vi "GrabToTrackerAndQueue(LostFramesSupport).vi"(0 "IMAQ Refnum in":refnum<k11>, 1 "Tracking enabled?":bool, 2 "Framerate":i32, 3 "QTrk Instance":T6, 4 "ROIs":cluster{"X":i32, "Y":i32}[](array[cluster]), 6 "stop":refnum<vi>, 7 "Type":T5, 8 "Send to queue?":bool, 9 "#ROI":i32, 10 "Output Queue":refnum<queue>, 12 "ResultManager":T4, 13 "ROI Size":cluster{"X":i32, "Y":i32}) -> ()   [LabVIEW 2011]
uses:
  qtrk/QTrkLVBinding/QTrkInstance.ctl
  Main/Typedefs/CmdEnum_CameraFrameType.ctl
  qtrk/QTrkLVBinding/ResultManagerInstance.ctl
  Main/Typedefs/CmdData_NewFrame.ctl
  <vilib>/vision/Image Controls.llb/IMAQ Image.ctl
  Main/Motors/MotorPosType.ctl
  Main/Typedefs/XYf.ctl
  qtrk/QTrkLVBinding/QTrkDLL.vi
  Main/GlobalVariables.vi
panel:
  out "Current Position":T1
  out "widths":u32[](array[numeric])
  out "Preloaded timestamps":u32[](array[numeric])
  in  "Stop2":bool
  in  "Show image?":bool
  out "Image":T3(plugin-control)
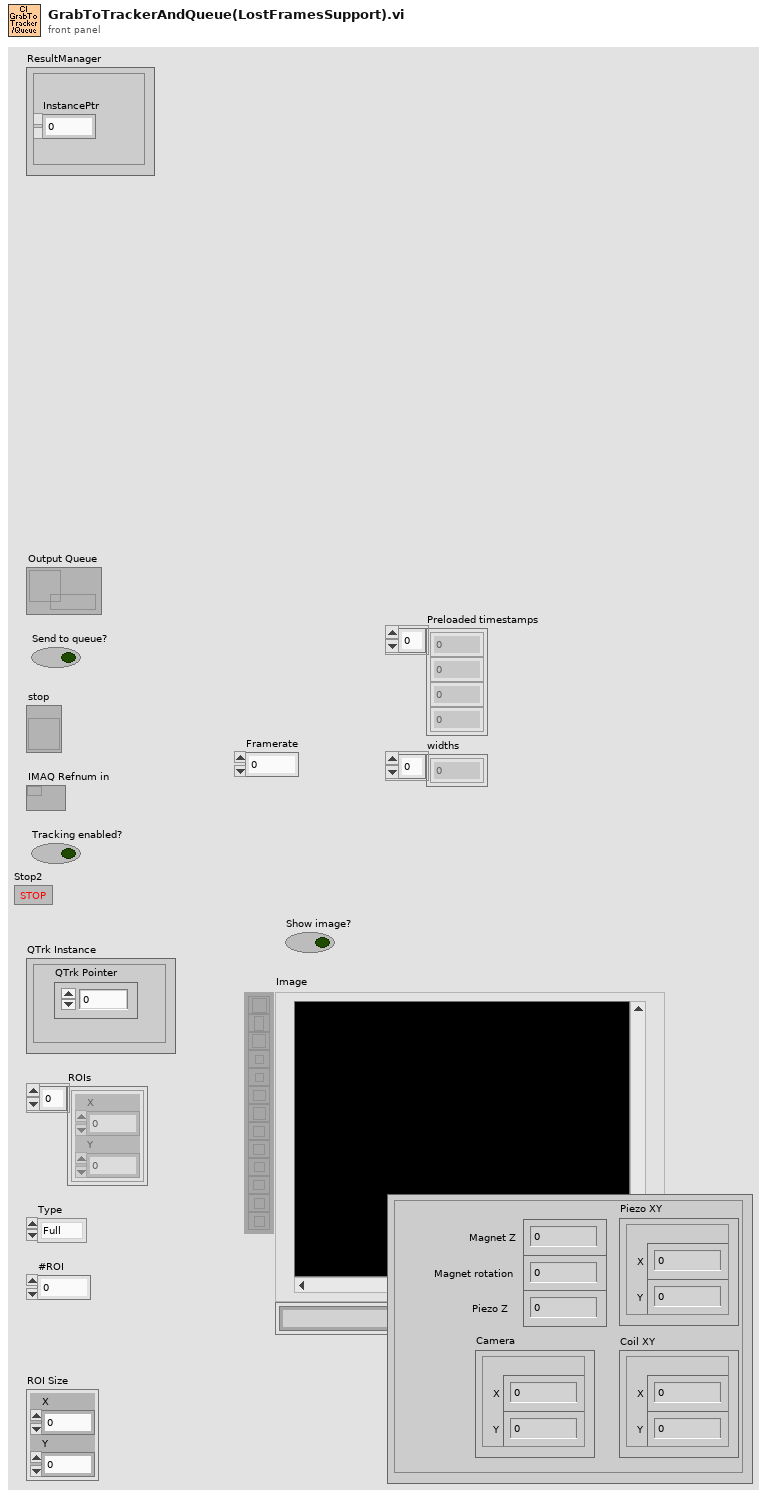
[diagram p1: front panel]
types:
  T1 = typedef "MotorPosType.ctl" = cluster{"Magnet Z":dbl, "Magnet rotation":dbl, "Camera":T2, "Piezo XY":T2, "Piezo Z":dbl, "Coil XY":T2}
  T2 = typedef "XYf.ctl" = cluster{"X":sgl, "Y":sgl}
  T3 = typedef "IMAQ Image.ctl" = refnum<image>
  T4 = typedef "ResultManagerInstance.ctl" = cluster{"InstancePtr":u64}
  T5 = typedef "CmdEnum_CameraFrameType.ctl" = enum16{"Full", "HardwareROI", "EndGrabMarker"}
  T6 = typedef "QTrkInstance.ctl" = cluster{"QTrk Pointer":u64}
  T7 = typedef "MotorStateType.ctl" = cluster{"Enabled?":bool, "Current Position":T1, "Update counter":i32}
  T8 = typedef "CmdData_NewFrame.ctl" = cluster{"Buffer Image":T3, "Frame #":i32, "Hardware ROI Index":i32, "Timestamp":dbl, "Type":T5}
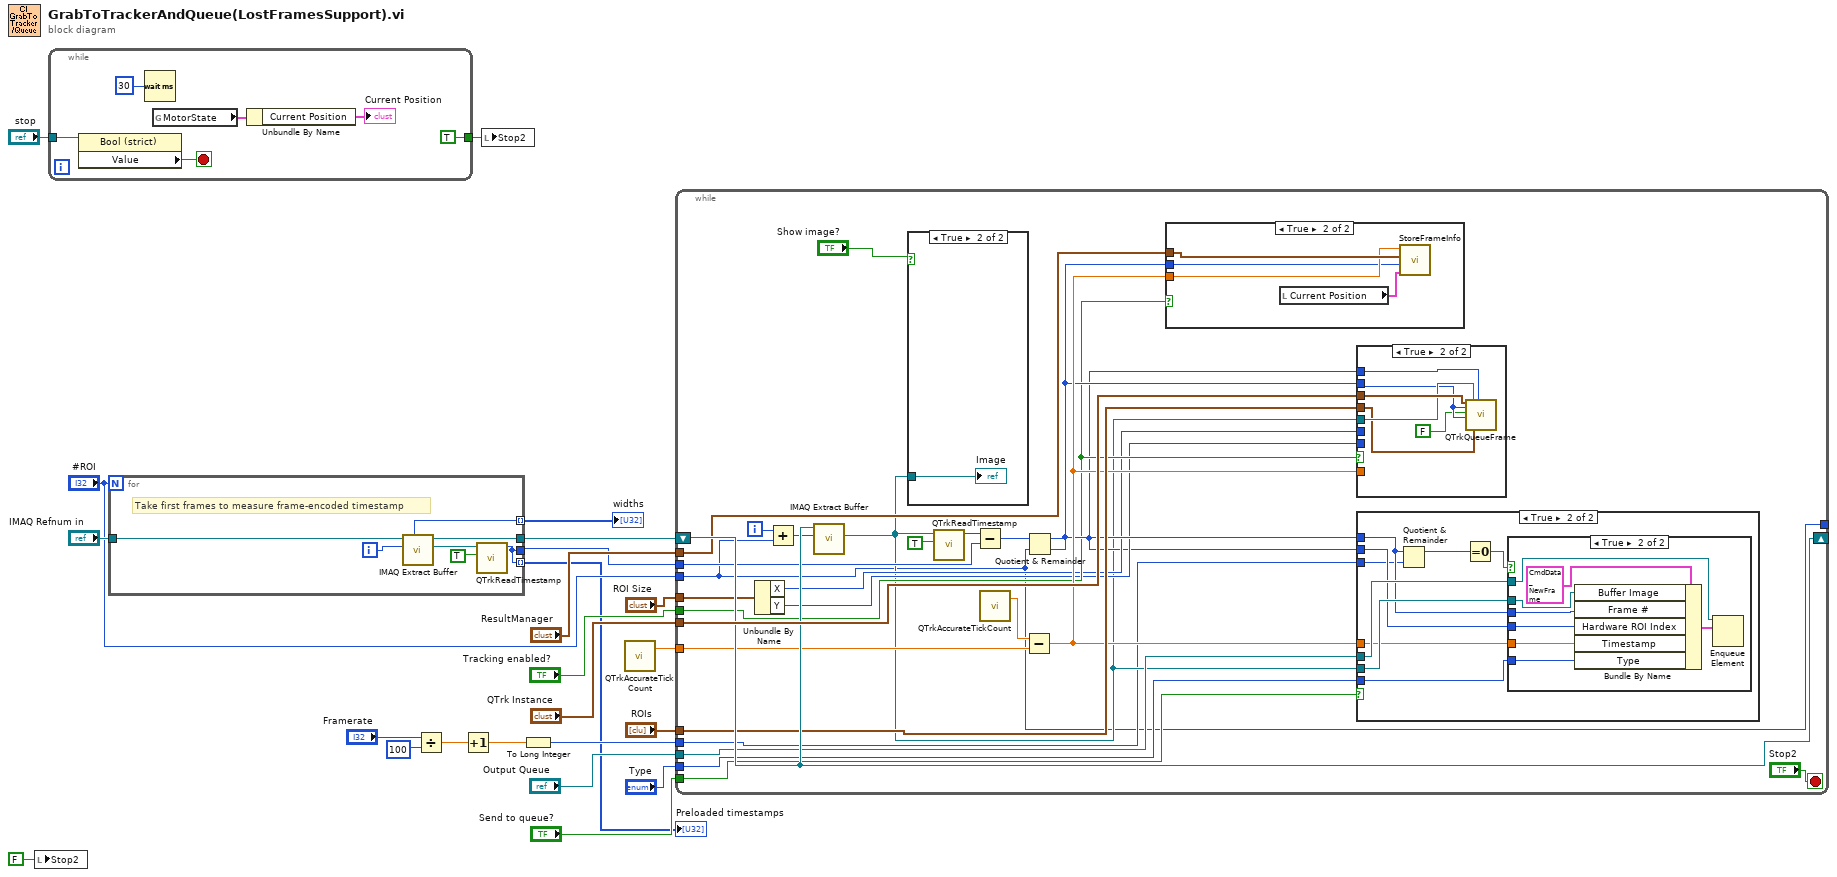
[diagram p0: block diagram]
diagram:
  n1 = local write "Stop2"(FALSE ("Stop2")) -> ()
  n2 = while {
    tunnel: "stop" -> [w28]
    tunnel: [TRUE ("Stop2")] -> w10
    stop <- w29 stop-if-true
    n3 = property on="Property Node" class="Bool (strict)"(reference=w28) -> ("Value"=w29:bool)  [unwired: 1 in, 2 out]
    n4 = Wait (ms)(milliseconds to wait=u32 30) -> ()  [unwired: 1 out]
    n5 = global read "GlobalVariables.vi" "MotorState"() -> (w25:T7)
    n6 = Unbundle By Name(w25) -> ("Current Position"=→"Current Position":T1)
  }
  n7 = for {
    N: "#ROI" -> [_]
    tunnel: "IMAQ Refnum in" -> [w35]
    tunnel: [w34] -> w13
    tunnel: [w32] -> w1
    tunnel: [w32] -> w3 mode=indexing
    tunnel: [w31] -> w2 mode=indexing
    i -> [w33]
    # "Take first frames to measure frame-encoded timestamp"
    n8 = call <vilib>:"IMAQ Extract Buffer.vi"("Buffer to extract"=w33, "IMAQ Session In"=w35) -> ("Image Out"=w36:T3, "IMAQ Session Out"=w34:refnum<k11>, "Actual Width"=w31:u32)  [unwired: 4 in, 3 out]
    n9 = call "QTrkReadTimestamp.vi"("Use QTrk code?"=TRUE, "Image"=w36) -> ("timestamp"=w32:u32)  [unwired: 9 in]
  }
  "Preloaded timestamps" <- w3
  "widths" <- w2
  n10 = Divide(x="Framerate", y=100) -> (x/y=w6:dbl)
  n11 = Increment(x=w6) -> (x+1=w5:dbl)
  n12 = local write "Stop2"(w10) -> ()
  n13 = To Long Integer(number=w5) -> (32bit integer=w4:i32)
  n14 = call "QTrkAccurateTickCount.vi"() -> ("tick count (ms)"=w15:dbl)  [unwired: 2 in, 1 out]
  n15 = while {
    tunnel: "Output Queue" -> [w57]
    shift-right: [w62] -> _
    shift-left: w13 -> [w62]
    tunnel: "QTrk Instance" -> [w63]
    tunnel: [w38] -> _
    tunnel: w15 -> [w60]
    tunnel: "ROIs" -> [w59]
    tunnel: "ResultManager" -> [w58]
    tunnel: "Type" -> [w55]
    tunnel: "Send to queue?" -> [w54]
    tunnel: w1 -> [w53]
    tunnel: "ROI Size" -> [w52]
    tunnel: "Tracking enabled?" -> [w50]
    tunnel: "#ROI" -> [w38]
    tunnel: w4 -> [w41]
    i -> [w39]
    stop <- "Stop2" stop-if-true
    n16 = Unbundle By Name(w52) -> ("X"=w49:i32, "Y"=w48:i32)
    n17 = Add(x=w39, y=w38) -> (x+y=w37:i32)
    n18 = call <vilib>:"IMAQ Extract Buffer.vi"("Buffer to extract"=w37, "IMAQ Session In"=w62) -> ("Image Out"=w43:T3)  [unwired: 4 in, 5 out]
    n19 = case shown="True" "Show image?" {
      tunnel: w43 -> [_ w64]
      frame False {
      }
      frame True {
        "Image" <- w64
      }
    }
    n20 = call "QTrkReadTimestamp.vi"("Use QTrk code?"=TRUE, "Image"=w43) -> ("timestamp"=w45:u32)  [unwired: 9 in]
    n21 = Subtract(x=w45, y=w53) -> (x-y=w47:u32)
    n22 = call "QTrkAccurateTickCount.vi"() -> ("tick count (ms)"=w61:dbl)  [unwired: 2 in, 1 out]
    n23 = Subtract(x=w61, y=w60) -> (x-y=w56:dbl)
    n24 = Quotient & Remainder(x=w47, y=w38) -> (x-y*floor(x/y)=w46:u32, floor(x/y)=w51:u32)
    n25 = case shown="True" w50 {
      tunnel: w58 -> [_ w91]
      tunnel: w56 -> [_ w90]
      tunnel: w51 -> [_ w89]
      frame False {
      }
      frame True {
        n26 = local read "Current Position"() -> (w88:T1)
        n27 = call "StoreFrameInfo.vi"("Current Position"=w88, "frame"=w89, "ResultManager"=w91, "Timestamp"=w90) -> ()  [unwired: 8 in]
      }
    }
    n28 = case shown="True" w50 {
      tunnel: w63 -> [_ w87]
      tunnel: w56 -> [_ _]
      tunnel: w59 -> [_ w83]
      tunnel: w49 -> [_ _]
      tunnel: w48 -> [_ _]
      tunnel: w51 -> [_ w84]
      tunnel: w46 -> [_ w85]
      tunnel: w43 -> [_ w86]
      frame False {
      }
      frame True {
        n29 = call "QTrkQueueFrame.vi"("QTrk Instance"=w87, "frame#"=w84, "Clear first 4 bytes in frame? (F)"=FALSE, "timestamp"=w84, "Image"=w86, "ROI Positions (corner-based)"=w83, "ZLUT Index offset (0)"=w85) -> ()  [unwired: 10 in, 3 out]
      }
    }
    n30 = case shown="True" w54 {
      tunnel: w57 -> [_ w73]
      tunnel: w43 -> [_ w72]
      tunnel: w56 -> [_ w71]
      tunnel: w55 -> [_ w70]
      tunnel: w51 -> [_ w68]
      tunnel: w46 -> [_ w69]
      tunnel: w41 -> [_ w67]
      frame False {
      }
      frame True {
        n31 = Quotient & Remainder(x=w68, y=w67) -> (x-y*floor(x/y)=w66:u32)  [unwired: 1 out]
        n32 = Equal To 0?(x=w66) -> (x = 0?=w65:bool)
        n33 = case shown="True" w65 {
          tunnel: w73 -> [_ w81]
          tunnel: w72 -> [_ w79]
          tunnel: w71 -> [_ w78]
          tunnel: w70 -> [_ w77]
          tunnel: w69 -> [_ w75]
          tunnel: w68 -> [_ w74]
          frame False {
          }
          frame True {
            n34 = Bundle By Name(cluster=T8 {"Buffer Image"=refnum, "Frame #"=0, "Hardware ROI Index"=0, "Timestamp"=0.0, "Type"=enum."Full"} ("element"), "Buffer Image"=w79, "Frame #"=w74, "Hardware ROI Index"=w75, "Timestamp"=w78, "Type"=w77) -> (w76:T8)
            n35 = Enqueue Element(queue=w81, element=w76) -> ()  [unwired: 2 in, 3 out]
          }
        }
      }
    }
  }
